vi "DAQANALOG_1.vi"() -> ()   [LabVIEW 2020, in "Acquisition.lvlib"]
uses:
  Acquisition.lvlib
  <vilib>/DAQmx/read.llb/DAQmx Read (Analog 1D Wfm NChan NSamp).vi
  <vilib>/DAQmx/miscellaneous.llb/DAQmx Fill In Error Info.vi
panel:
  out "data":waveform(dbl)[](graph)
  in  "stop":bool
  in  "rate":dbl=1000.0 format="%0.2f"
  in  "error in":errorcluster
  in  "number of samples":i32=1000
  in  "Canales":tag[](array[tag])
  in  "DAQ Board Name":tag
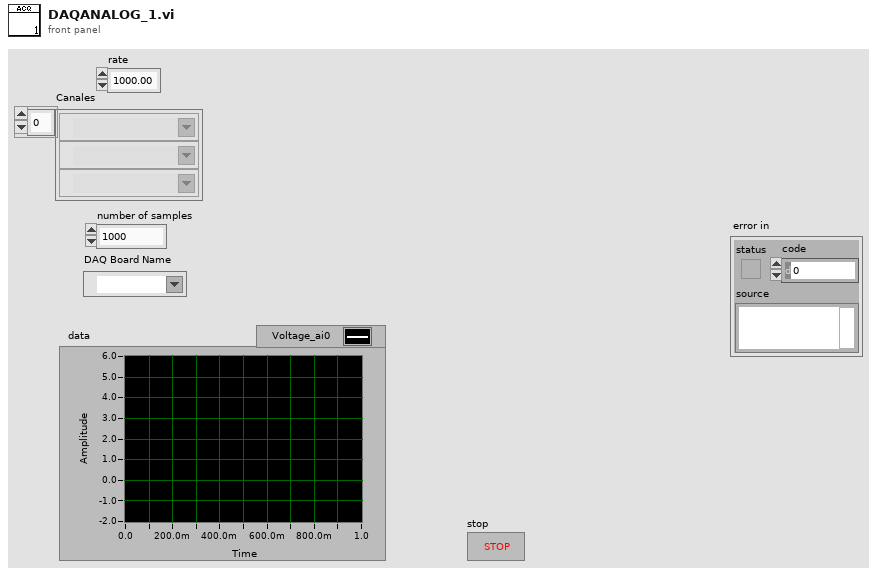
[diagram p1: front panel]
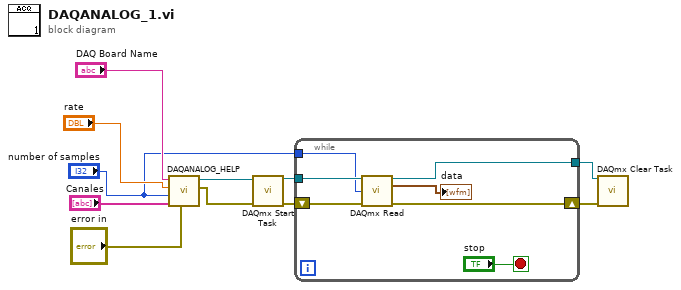
[diagram p0: block diagram]
diagram:
  n1 = call "DAQANALOG_HELP.vi"("error in"="error in", "Canales"="Canales", "number of samples"="number of samples", "Frecuencia de muestreo"="rate", "DAQ Board Name"="DAQ Board Name") -> ("error out"=w6:errorcluster, "task out"=w7:refnum<k21>)  [unwired: 5 in]
  n2 = call <vilib>:"DAQmx Start Task.vi"("task/channels in"=w7, "error in"=w6) -> ("task out"=w11:refnum<k21>, "error out"=w10:errorcluster)  [unwired: 12 in]
  n3 = while {
    tunnel: w11 -> [w18]
    tunnel: [w15] -> w8
    shift-right: [w14] -> w9
    shift-left: w10 -> [w17]
    tunnel: "number of samples" -> [w12]
    stop <- "stop" stop-if-true
    n4 = call-poly <vilib>:"DAQmx Read.vi"("task/channels in"=w18, "number of samples per channel"=w12, "error in"=w17) -> ("task out"=w15:refnum<k21>, "data"=→"data":waveform(dbl)[], "error out"=w14:errorcluster)  [unwired: 10 in]
  }
  n5 = call <vilib>:"DAQmx Clear Task.vi"("task in"=w8, "error in"=w9) -> ()  [unwired: 13 in, 1 out]
